vi "太阳能控制器MPPT12.vi"() -> ()   [LabVIEW 2016, in "环境动力监测库.lvlib"]
uses:
  <vilib>/Utility/miscctls.llb/LVPointTypeDef.ctl
  <vilib>/Utility/config.llb/NI_LVConfig.lvlib
  <vilib>/ptbypt/NI_PtbyPt.lvlib
panel:
  out "x+1":u32
  in  "解除告警":bool
  out "串口":string
  in  "串口启用":bool
  in  "MPPT-12 串口":refnum<visa-resource-name> caption="MPPT-12"
  out "状态":string
  out "充放电信息":T1 caption="充放电信息_KWH" {"总累计充电量" format="%.2f"; "当年累计充电量" format="%.2f"; "当月累计充电量" format="%.2f"; "当日累计充电量" format="%.2f"; "当年累计用电量" format="%.2f"; "当月累计用电量" format="%.2f"; "当日累计用电量" format="%.2f"}
  out "通信":bool=TRUE
  out "控制器信息":cluster{"设备温度":dbl}
  out "直流负载信息":cluster{"负载电压":dbl, "负载电流":dbl, "负载功率":dbl}
  out "蓄电池信息":T2
  out "阵列信息":cluster{"阵列电压":dbl, "阵列电流":dbl, "发电功率":dbl}
  # "太阳能控制器MPPT-12"
  # "kW·h"
  # "kW·h"
  # "kW·h"
  # "kW·h"
  # "kW·h"
  # "kW·h"
  # "kW·h"
  # "kW·h"
  # "℃"
  # "V"
  # "A"
  # "W"
  # "V"
  # "A"
  # "V"
  # "V"
  # "℃"
  # "%"
  # "V"
  # "A"
  # "W"
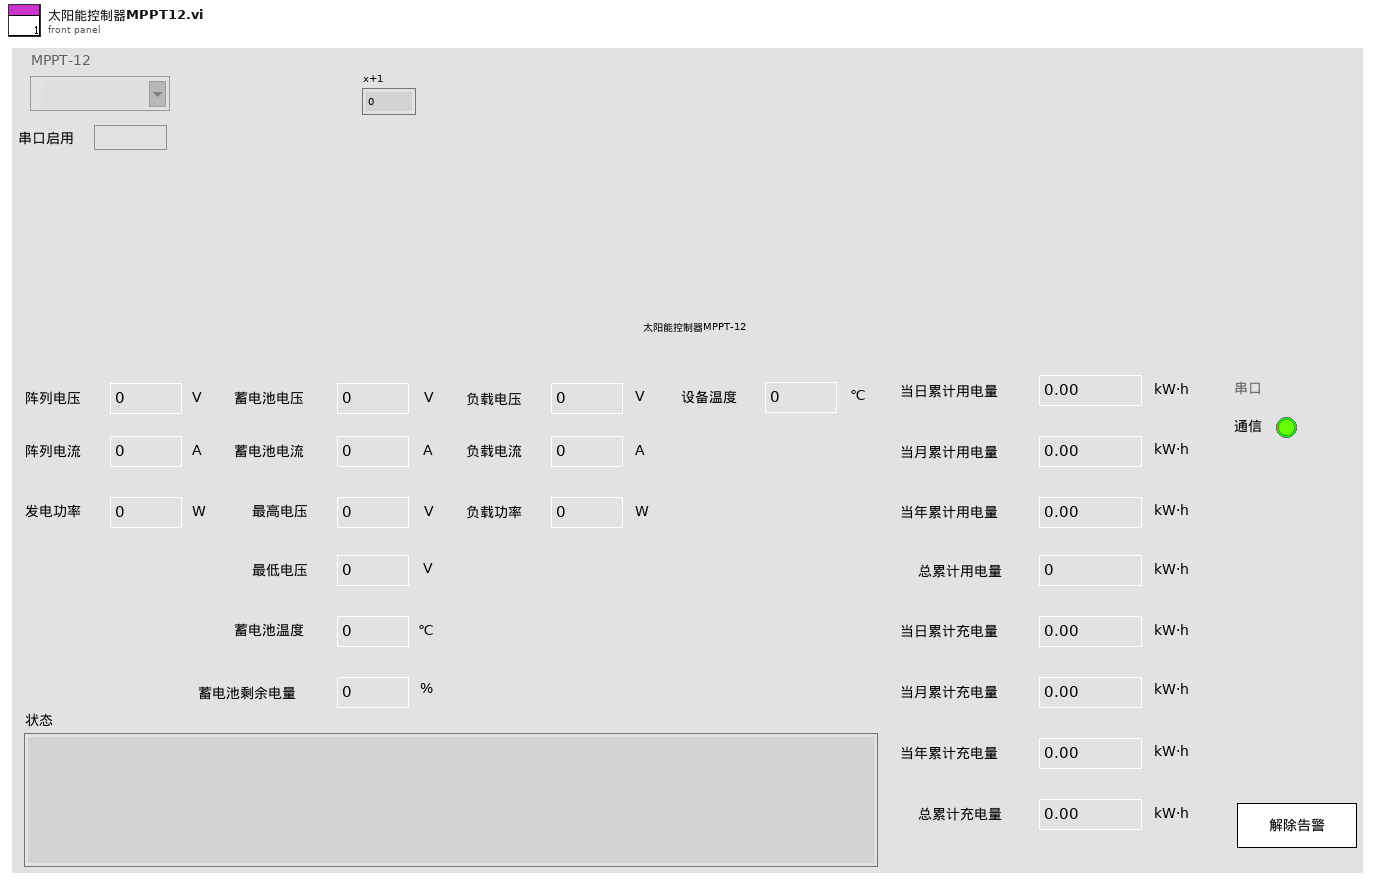
[diagram p1: front panel]
types:
  T1 = cluster{"当日累计用电量":sgl, "当月累计用电量":sgl, "当年累计用电量":sgl, "总累计用电量":sgl, "当日累计充电量":sgl, "当月累计充电量":sgl, "当年累计充电量":sgl, "总累计充电量":sgl}
  T2 = cluster{"蓄电池电压":dbl, "蓄电池电流":dbl, "最高电压":dbl, "最低电压":dbl, "蓄电池温度":dbl, "蓄电池剩余电量":dbl}
  T3 = typedef "LVPointTypeDef.ctl" = cluster{"Horizontal":i16, "Vertical":i16}
  T4 = cluster{"漏水监测输出":cluster{"漏水监测告警":bool, "告警内容":string}, "门禁监测输出":cluster{"门禁监测告警":bool, "告警内容":string}, "门禁监测输出2":cluster{"门禁监测告警":bool, "告警内容":string}, "温湿度监测输出":cluster{"温湿度监测告警":bool, "告警内容":string}, "烟雾监测输出":cluster{"烟雾监测告警":bool, "告警内容":string}, "空调监测输出":cluster{"空调监测告警":bool, "告警内容":string}, "自动重合闸输出":cluster{"自动重合闸告警":bool, "告警内容":string}, "红外入侵输出":cluster{"红外入侵告警":bool, "告警内容":string}, "振动输出":cluster{"振动告警":bool, "告警内容":string}, "UPS输出":cluster{"UPS告警":bool, "告警内容":string}, "蓄电池输出":cluster{"蓄电池告警":bool, "告警内容":string}, "蓄电池输出2":cluster{"蓄电池告警":bool, "告警内容":string}, "GPS输出":cluster{"定位告警":bool, "告警内容":string}, "北斗输出":cluster{"定位告警":bool, "告警内容":string}, "气象输出":cluster{"气象告警":bool, "告警内容":string}, "废液输出":cluster{"废液告警":bool, "告警内容":string}, "废液输出2":cluster{"废液告警":bool, "告警内容":string}}
  T5 = cluster{"时间":timestamp, "阵列电压_V":dbl, "阵列电流_A":dbl, "发电功率_W":dbl, "蓄电池电压_V":dbl, "蓄电池电流_A":dbl, "最高电压_V":dbl, "最低电压_A":dbl, "蓄电池温度_℃":dbl, "蓄电池剩余电量_%":dbl, "负载电压_V":dbl, "负载电流_A":dbl, "负载功率_W":dbl, "设备温度_℃":dbl, "当日累计用电量_KWH":dbl, "当月累计用电量_KWH":dbl, "当年累计用电量_KWH":dbl, "总累计用电量_KWH":dbl, "当日累计充电量_KWH":dbl, "当月累计充电量_KWH":dbl, "当年累计充电量_KWH":dbl, "总累计充电量_KWH":dbl}
  T6 = typedef "LVDateTimeRec.ctl" = cluster{"秒数的小数部分":dbl, "秒":i32, "分":i32, "时":i32, "日":i32, "月":i32, "年":i32, "天数（周）":i32, "天数（年）":i32, "DST":i32}
  T7 = cluster{"市电":cluster{"状态":bool, "电压:":u16, "电流：":dbl, "详情  ":bool}, "UPS":cluster{"状态":bool, "输入电压:":sgl, "输出电压:":sgl, "电池电量:":u8, "电量":u16, "详情  ":bool}, "蓄电池12V":cluster{"状态":bool, "电压:":sgl, "电流:":sgl, "电池电量:":u8, "电量":u16, "详情  ":bool, "充电":bool, "负载":bool}, "蓄电池24V":cluster{"状态":bool, "电压:":sgl, "电流:":sgl, "电池电量:":u8, "电量":u16, "详情  ":bool, "充电":bool, "负载":bool}}
  T8 = cluster{"状态":cluster{"蓄电池状态":string, "阵列状态":string, "充电状态":string, "负载状态":string, "设备状态":string}, "充放电信息":cluster{"当日累计用电量":sgl, "当月累计用电量":sgl, "当年累计用电量":sgl, "总累计用电量":sgl, "当日累计充电量":sgl, "当月累计充电量":sgl, "当年累计充电量":sgl, "总累计充电量":sgl}, "控制器信息":cluster{"设备温度℃":dbl}, "蓄电池信息":cluster{"蓄电池电压V":dbl, "蓄电池电流A":dbl, "最高电压V":dbl, "最低电压A":dbl, "蓄电池温度℃":dbl, "蓄电池剩余电量%":dbl}, "阵列信息":cluster{"阵列电压V":dbl, "阵列电流A":dbl, "发电功率W":dbl}, "直流负载信息":cluster{"负载电压V":dbl, "负载电流A":dbl, "负载功率W":dbl}, "error out":errorcluster}
  T9 = enum32{"Bad", "Idle", "Run top level", "Running"}
  T10 = typedef "NI_LVConfig.lvlib/Config Data RefNum.ctl" = refnum<k1>
  T11 = enum8{"Enabled", "Disabled", "Disabled and Grayed Out"}
  T12 = cluster{"蓄电池电压V":dbl, "蓄电池电流A":dbl, "最高电压V":dbl, "最低电压A":dbl, "蓄电池温度℃":dbl, "蓄电池剩余电量%":dbl}
  T13 = cluster{"蓄电池状态":string, "阵列状态":string, "充电状态":string, "负载状态":string, "设备状态":string}
  T14 = cluster{"baud rate (bps)":u32, "stop bits":u16, "parity":u16, "flow control":u16, "timeout":u32, "retries":i32}
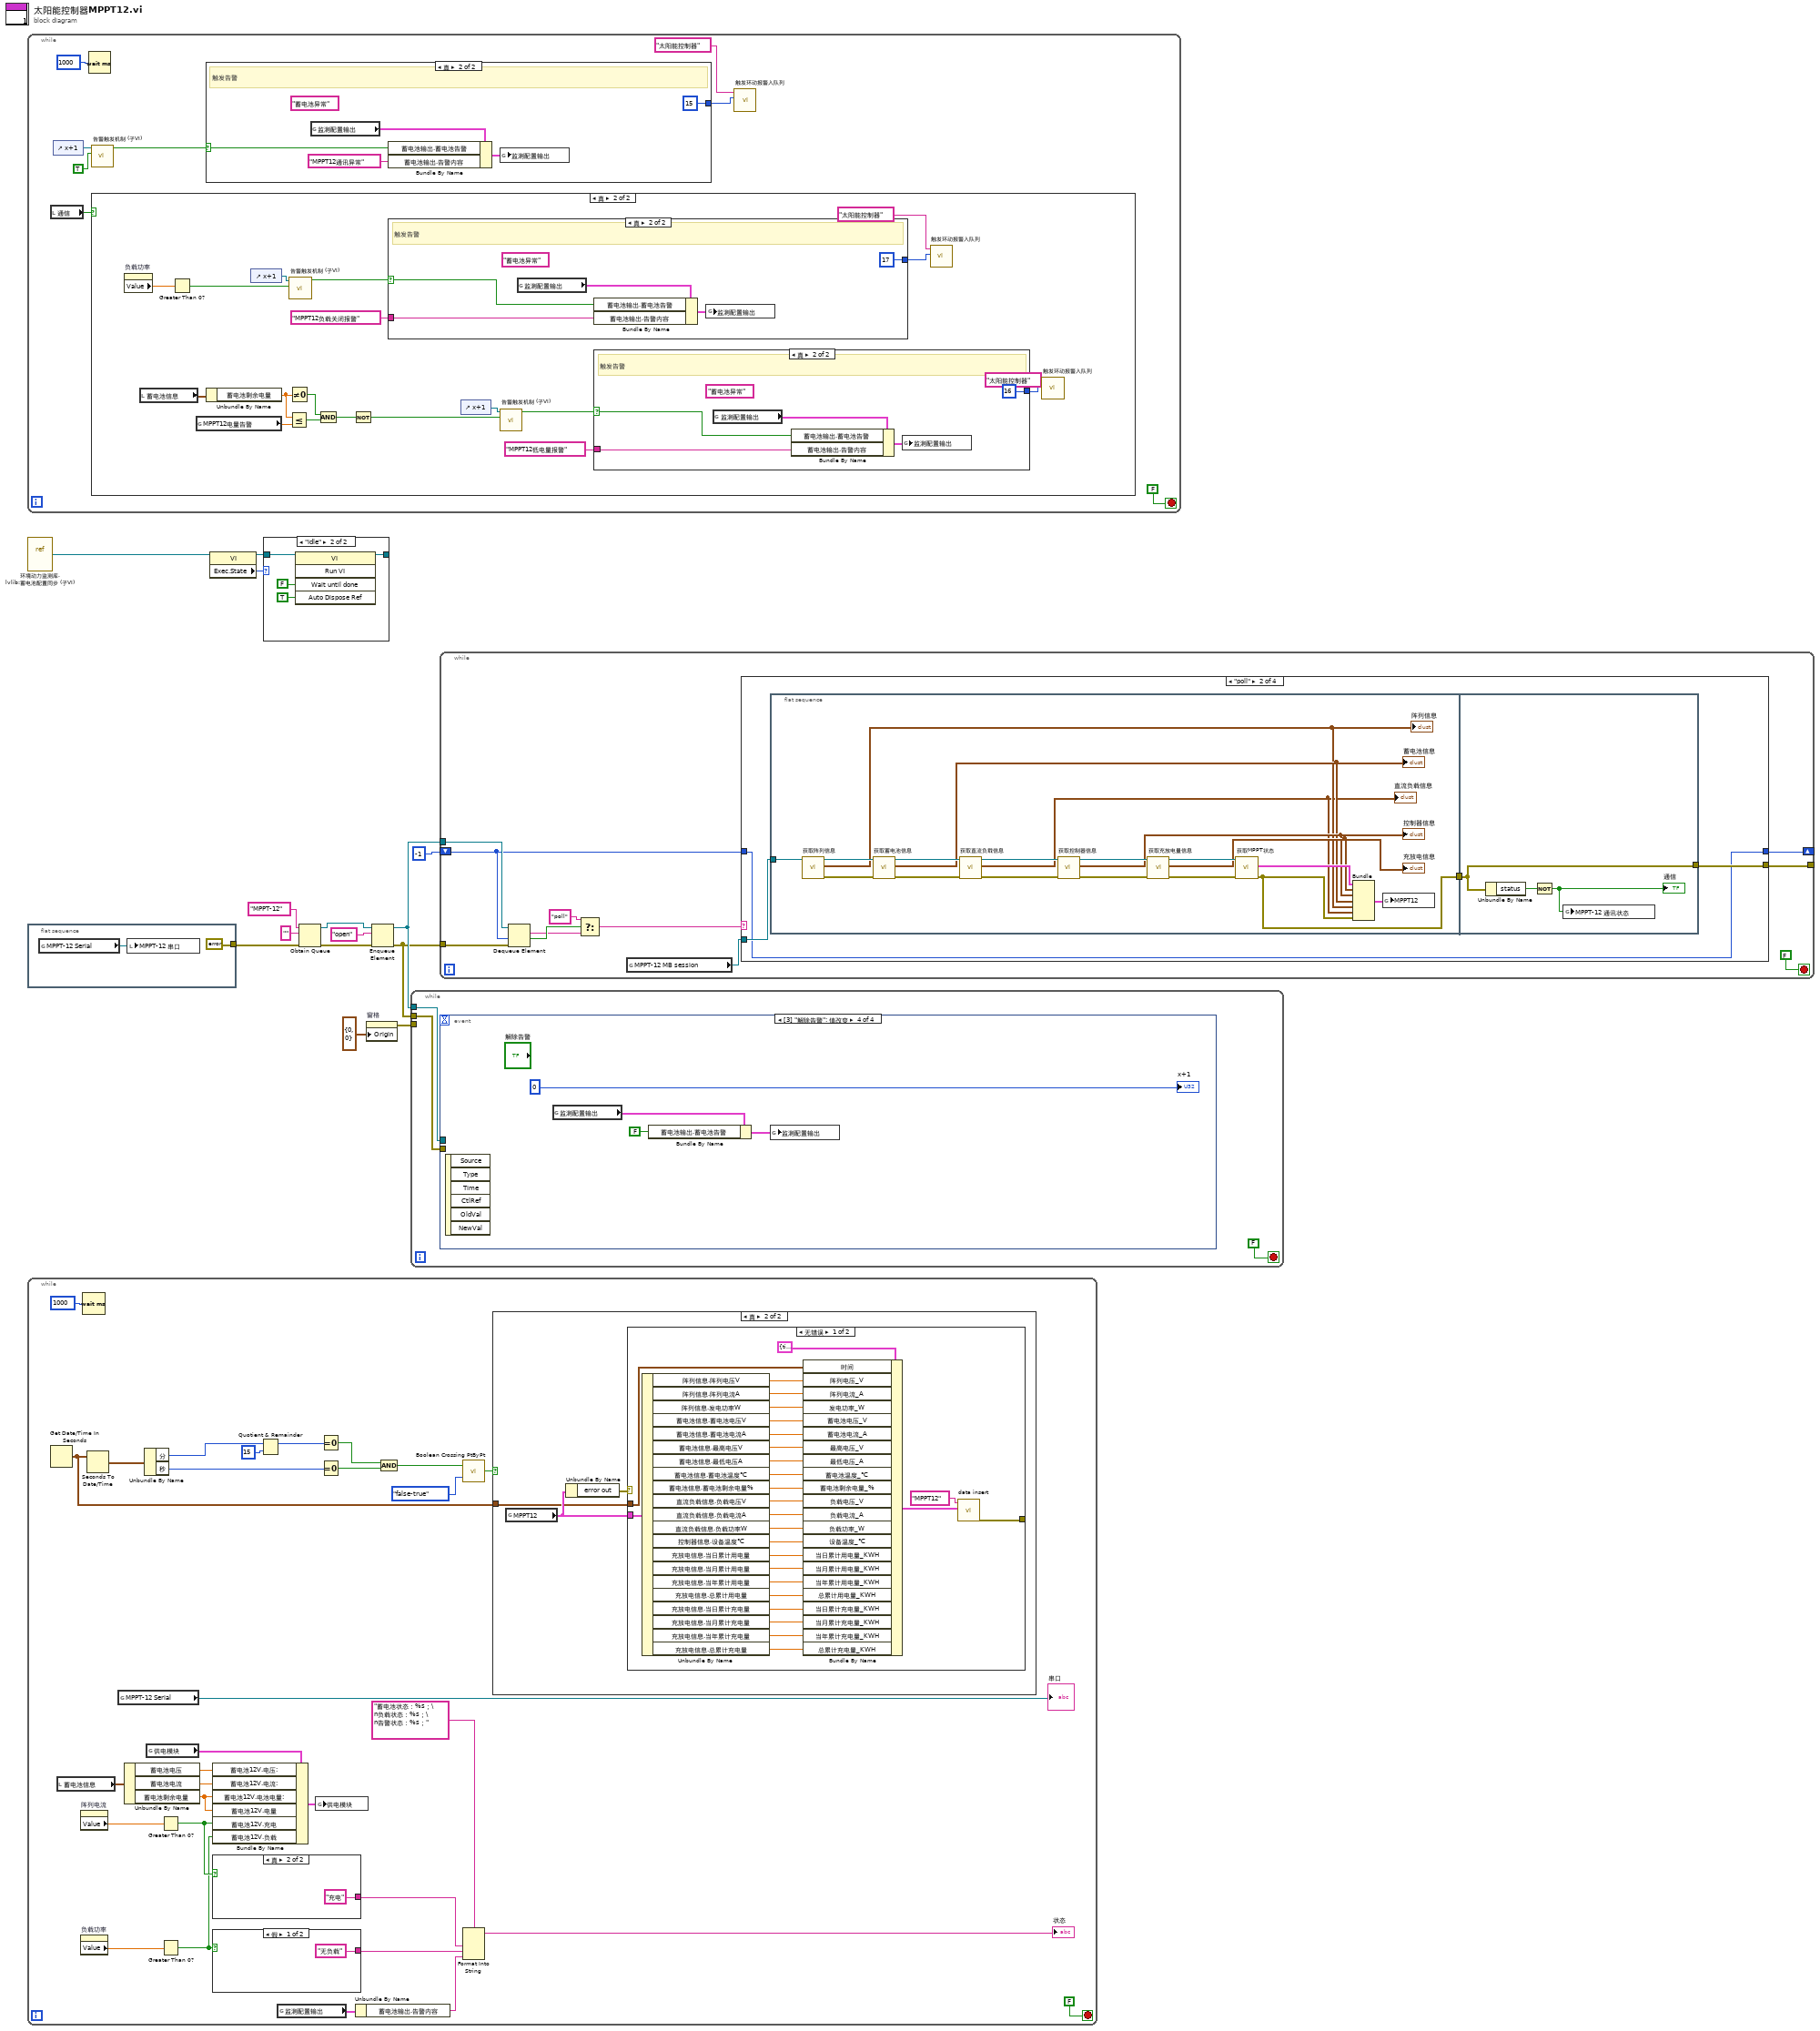
[diagram p0: block diagram]
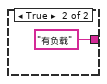
[diagram p7: hidden frame]
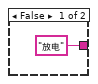
[diagram p8: hidden frame]
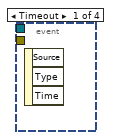
[diagram p11: hidden frame]
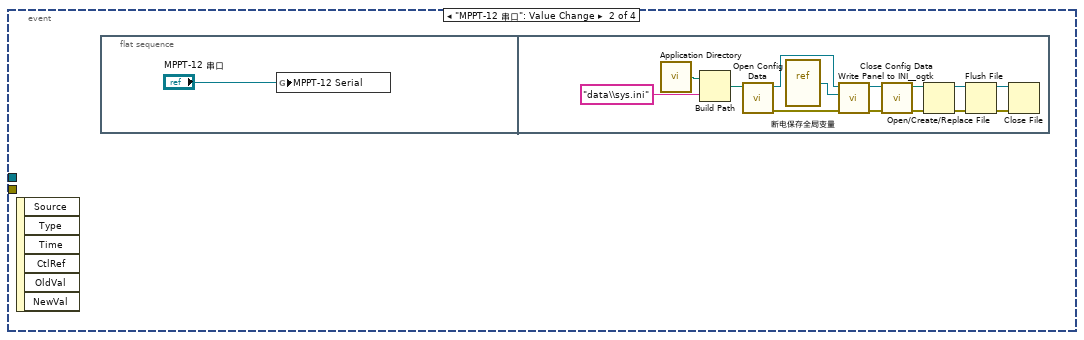
[diagram p12: hidden frame]
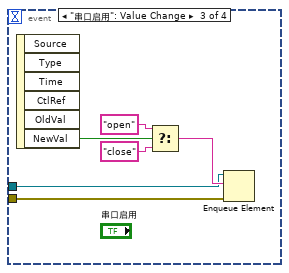
[diagram p13: hidden frame]
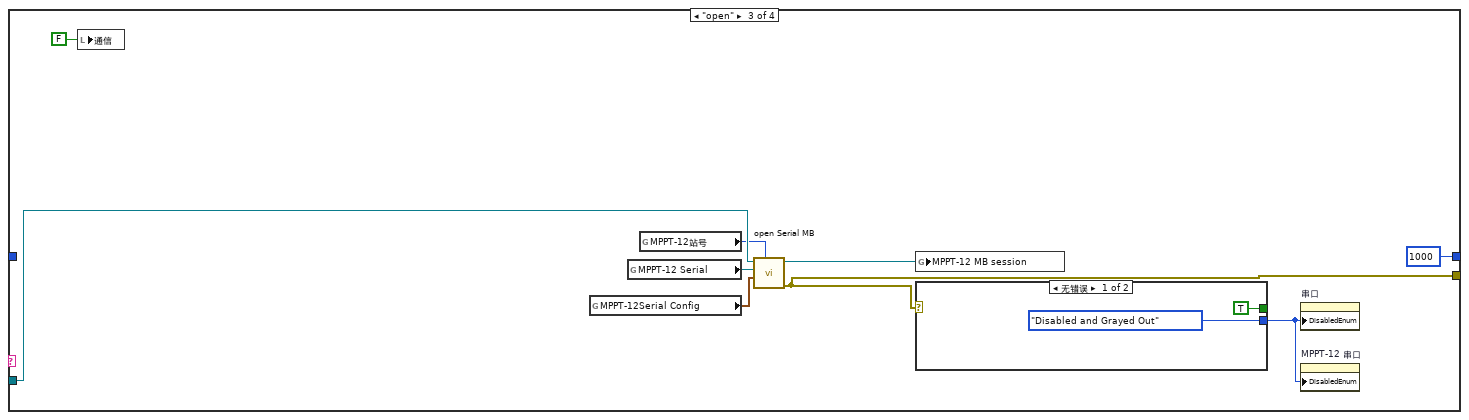
[diagram p15: hidden frame]
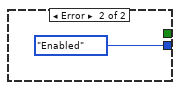
[diagram p16: hidden frame]
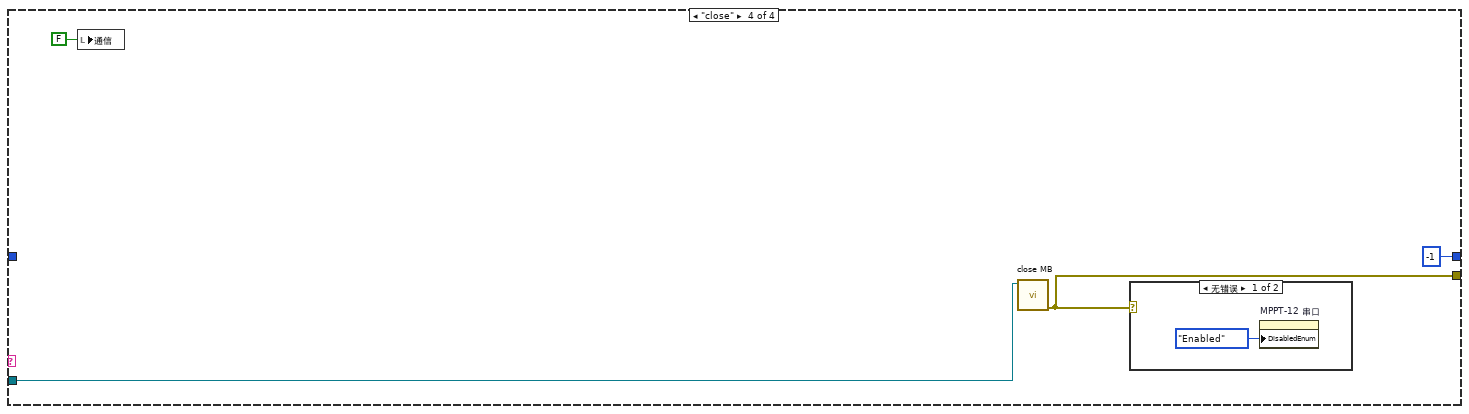
[diagram p17: hidden frame]
diagram:
  n1 = while {
    stop <- FALSE stop-if-true
    n2 = local read "通信"() -> (w20:bool)
    n3 = control-ref of="x+1"() -> (w19:refnum<vi>)
    n4 = Wait (ms)(milliseconds to wait=u32 1000 ("等待时间（毫秒）")) -> ()  [unwired: 1 out]
    n5 = call "告警触发机制 (子VI).vi"("状态输出"=TRUE, "Digital输入"=w19) -> ("触发告警"=w18:bool)  [unwired: 8 in, 1 out]
    n6 = case shown="真" w20 {
      frame False {
      }
      frame True {
        n7 = property on="负载功率" class="DigNum (严格)"() -> ("Value"=w36:dbl)  [unwired: 2 in, 2 out]
        n8 = local read "蓄电池信息"() -> (w46:T2)
        n9 = Greater Than 0?(x=w36) -> (x > 0?=w34:bool)
        n10 = global read "断电保存全局变量.vi" "MPPT12电量告警"() -> (w45:dbl)
        n11 = Unbundle By Name(w46) -> ("蓄电池剩余电量"=w39:dbl)
        n12 = control-ref of="x+1"() -> (w35:refnum<vi>)
        n13 = Less Or Equal?(x=w39, y=w45) -> (x <= y?=w40:bool)
        n14 = Not Equal To 0?(x=w39) -> (x != 0?=w38:bool)
        n15 = call "告警触发机制 (子VI).vi"("状态输出"=w34, "Digital输入"=w35) -> ("触发告警"=w32:bool)  [unwired: 8 in, 1 out]
        n16 = And(x=w38, y=w40) -> (x .and. y?=w37:bool)
        n17 = Not(x=w37) -> (.not. x?=w43:bool)
        n18 = case shown="真" w32 {
          selector: w32 -> [_ w51]
          tunnel: "MPPT12负载关闭报警" ("设备") -> [_ w48]
          tunnel: [_ 17 ("code")] -> w29
          frame False {
          }
          frame True {
            (unwired) "蓄电池异常" ("设备")
            # "触发告警"
            n19 = global read "内部交互全局变量.vi" "监测配置输出"() -> (w50:T4)
            n20 = Bundle By Name(cluster=w50, "蓄电池输出.蓄电池告警"=w51, "蓄电池输出.告警内容"=w48) -> (w49:T4)
            n21 = global write "内部交互全局变量.vi" "监测配置输出"(w49) -> ()
          }
        }
        n22 = control-ref of="x+1"() -> (w41:refnum<vi>)
        n23 = call "告警触发机制 (子VI).vi"("状态输出"=w43, "Digital输入"=w41) -> ("触发告警"=w42:bool)  [unwired: 8 in, 1 out]
        n24 = case shown="真" w42 {
          selector: w42 -> [_ w56]
          tunnel: "MPPT12低电量报警" ("设备") -> [_ w53]
          tunnel: [_ 16 ("code")] -> w31
          frame False {
          }
          frame True {
            (unwired) "蓄电池异常" ("设备")
            # "触发告警"
            n25 = global read "内部交互全局变量.vi" "监测配置输出"() -> (w55:T4)
            n26 = Bundle By Name(cluster=w55, "蓄电池输出.蓄电池告警"=w56, "蓄电池输出.告警内容"=w53) -> (w54:T4)
            n27 = global write "内部交互全局变量.vi" "监测配置输出"(w54) -> ()
          }
        }
        n28 = call "触发环动报警入队列.vi"("code"=w29, "元器件"="太阳能控制器") -> ()  [unwired: 10 in]
        n29 = call "触发环动报警入队列.vi"("code"=w31, "元器件"="太阳能控制器") -> ()  [unwired: 10 in]
      }
    }
    n30 = case shown="真" w18 {
      selector: w18 -> [_ w27]
      tunnel: [_ 15 ("code")] -> w15
      frame False {
      }
      frame True {
        (unwired) "蓄电池异常" ("设备")
        # "触发告警"
        n31 = global read "内部交互全局变量.vi" "监测配置输出"() -> (w26:T4)
        n32 = Bundle By Name(cluster=w26, "蓄电池输出.蓄电池告警"=w27, "蓄电池输出.告警内容"="MPPT12通讯异常" ("报警内容")) -> (w25:T4)
        n33 = global write "内部交互全局变量.vi" "监测配置输出"(w25) -> ()
      }
    }
    n34 = call "触发环动报警入队列.vi"("code"=w15, "元器件"="太阳能控制器") -> ()  [unwired: 10 in]
  }
  n35 = vi-ref "环境动力监测库.lvlib:蓄电池配置同步 (子VI).vi"() -> (w2:refnum<vi>)
  n36 = flat-sequence {
    tunnel: [errorcluster {"status"=FALSE, "code"=0, "source"=""} ("error out")] -> w1
    frame #0 {
      n37 = global read "断电保存全局变量.vi" "MPPT-12 Serial"() -> (w58:refnum<visa-resource-name>)
      n38 = local write "MPPT-12 串口"(w58) -> ()
    }
  }
  n39 = while {
    stop <- FALSE stop-if-true
    n40 = Get Date/Time In Seconds() -> (seconds since 1Jan1904=w76:timestamp)
    n41 = local read "蓄电池信息"() -> (w72:T2)
    n42 = property on="阵列电流" class="DigNum (严格)"() -> ("Value"=w67:dbl)  [unwired: 2 in, 2 out]
    n43 = property on="负载功率" class="DigNum (严格)"() -> ("Value"=w63:dbl)  [unwired: 2 in, 2 out]
    n44 = Wait (ms)(milliseconds to wait=u32 1000 ("等待时间（毫秒）")) -> ()  [unwired: 1 out]
    n45 = Seconds To Date/Time(time stamp (now)=w76) -> (date time rec=w86:T6)  [unwired: 1 in]
    n46 = global read "断电保存全局变量.vi" "MPPT-12 Serial"() -> (→"串口":refnum<visa-resource-name>)
    n47 = Unbundle By Name(w72) -> ("蓄电池电压"=w71:dbl, "蓄电池电流"=w70:dbl, "蓄电池剩余电量"=w69:dbl)
    n48 = Unbundle By Name(w86) -> ("分"=w85:i32, "秒"=w82:i32)
    n49 = global read "内部交互全局变量.vi" "供电模块"() -> (w74:T7)
    n50 = Greater Than 0?(x=w67) -> (x > 0?=w64:bool)
    n51 = Greater Than 0?(x=w63) -> (x > 0?=w59:bool)
    n52 = Bundle By Name(cluster=w74, "蓄电池12V.电压:"=w71, "蓄电池12V.电流:"=w70, "蓄电池12V.电池电量:"=w69, "蓄电池12V.电量"=w69, "蓄电池12V.充电"=w64, "蓄电池12V.负载"=w59) -> (w73:T7)
    n53 = case shown="真" w64 {
      tunnel: ["放电" "充电"] -> w66
      frame False {
      }
      frame True {
      }
    }
    n54 = case shown="假" w59 {
      tunnel: ["无负载" "有负载"] -> w62
      frame False {
      }
      frame True {
      }
    }
    n55 = Quotient & Remainder(x=w85, y=15) -> (x-y*floor(x/y)=w83:i32)  [unwired: 1 out]
    n56 = global read "内部交互全局变量.vi" "监测配置输出"() -> (w61:T4)
    n57 = global write "内部交互全局变量.vi" "供电模块"(w73) -> ()
    n58 = Equal To 0?(x=w83) -> (x = 0?=w81:bool)
    n59 = Equal To 0?(x=w82) -> (x = 0?=w80:bool)
    n60 = Unbundle By Name(w61) -> ("蓄电池输出.告警内容"=w60:string)
    n61 = And(x=w81, y=w80) -> (x .and. y?=w79:bool)
    n62 = call <vilib>:"Boolean Crossing PtByPt.vi"("direction"=enum16{"either", "false-true", "true-false"}."false-true", "input"=w79) -> ("crossing"=w77:bool)  [unwired: 1 in]
    n63 = Format Into String(format string="蓄电池状态：%s；\n负载状态：%s；\n告警状态：%s；" ("格式字符串"), w66, w62, w60) -> (resulting string=→"状态":string)  [unwired: 2 in, 1 out]
    n64 = case shown="真" w77 {
      tunnel: w76 -> [_ w93]
      frame False {
      }
      frame True {
        n65 = global read "太阳能控制器全局.vi" "MPPT12"() -> (w94:T8)
        n66 = Unbundle By Name(w94) -> ("error out"=w95:errorcluster)
        n67 = case shown="无错误" w95 {
          tunnel: w94 -> [w100 _]
          tunnel: w93 -> [w99 _]
          tunnel: [w96 _] -> _
          frame No Error {
            n68 = Unbundle By Name(w100) -> ("阵列信息.阵列电压V"=w102:dbl, "阵列信息.阵列电流A"=w103:dbl, "阵列信息.发电功率W"=w104:dbl, "蓄电池信息.蓄电池电压V"=w105:dbl, "蓄电池信息.蓄电池电流A"=w106:dbl, "蓄电池信息.最高电压V"=w107:dbl, "蓄电池信息.最低电压A"=w108:dbl, "蓄电池信息.蓄电池温度℃"=w109:dbl, "蓄电池信息.蓄电池剩余电量%"=w110:dbl, "直流负载信息.负载电压V"=w111:dbl, "直流负载信息.负载电流A"=w112:dbl, "直流负载信息.负载功率W"=w113:dbl, "控制器信息.设备温度℃"=w114:dbl, "充放电信息.当日累计用电量"=w115:sgl, "充放电信息.当月累计用电量"=w116:sgl, "充放电信息.当年累计用电量"=w117:sgl, "充放电信息.总累计用电量"=w118:sgl, "充放电信息.当日累计充电量"=w119:sgl, "充放电信息.当月累计充电量"=w120:sgl, "充放电信息.当年累计充电量"=w121:sgl, "充放电信息.总累计充电量"=w122:sgl)
            n69 = Bundle By Name(cluster=T5 {"时间"=timestamp(0 s since 1904-01-01), "阵列电压_V"=0.0, "阵列电流_A"=0.0, "发电功率_W"=0.0, "蓄电池电压_V"=0.0, "蓄电池电流_A"=0.0, "最高电压_V"=0.0, "最低电压_A"=0.0, "蓄电池温度_℃"=0.0, "蓄电池剩余电量_%"=0.0, "负载电压_V"=0.0, "负载电流_A"=0.0, "负载功率_W"=0.0, "设备温度_℃"=0.0, "当日累计用电量_KWH"=0.0, "当月累计用电量_KWH"=0.0, "当年累计用电量_KWH"=0.0, "总累计用电量_KWH"=0.0, "当日累计充电量_KWH"=0.0, "当月累计充电量_KWH"=0.0, "当年累计充电量_KWH"=0.0, "总累计充电量_KWH"=0.0} ("data in"), "时间"=w99, "阵列电压_V"=w102, "阵列电流_A"=w103, "发电功率_W"=w104, "蓄电池电压_V"=w105, "蓄电池电流_A"=w106, "最高电压_V"=w107, "最低电压_A"=w108, "蓄电池温度_℃"=w109, "蓄电池剩余电量_%"=w110, "负载电压_V"=w111, "负载电流_A"=w112, "负载功率_W"=w113, "设备温度_℃"=w114, "当日累计用电量_KWH"=w115, "当月累计用电量_KWH"=w116, "当年累计用电量_KWH"=w117, "总累计用电量_KWH"=w118, "当日累计充电量_KWH"=w119, "当月累计充电量_KWH"=w120, "当年累计充电量_KWH"=w121, "总累计充电量_KWH"=w122) -> (w98:T5)
            n70 = call "data insert.vi"("data in"=w98, "table"="MPPT12") -> ("error out"=w96:errorcluster)  [unwired: 9 in]
          }
          frame Error {
          }
        }
      }
    }
  }
  n71 = property class="VI"(reference=w2) -> (reference out=w3:refnum<vi>, "Exec.State"=w4:T9)  [unwired: 1 in, 1 out]
  n72 = case shown="\"Idle\"" w4 {
    tunnel: w3 -> [w123 w125]
    tunnel: [w123 w124] -> _
    frame "Bad", Default {
    }
    frame "Idle" {
      n73 = invoke class="VI" method="Run VI"(reference=w125, "Wait until done"=FALSE ("结束前等待"), "Auto Dispose Ref"=TRUE ("自动销毁引用")) -> (reference out=w124:refnum<vi>)  [unwired: 2 in, 4 out]
    }
  }
  n74 = Obtain Queue(name (unnamed)="MPPT-12" ("名称（未命名）"), element data type="", error in (no error)=w1) -> (queue out=w8:refnum<queue>, error out=w7:errorcluster)  [unwired: 2 in, 1 out]
  n75 = property on="窗格" class="Pane"("Origin"=T3 {"Horizontal"=0, "Vertical"=0} ("原点")) -> (error out=w12:errorcluster)  [unwired: 2 in, 1 out]
  n76 = Enqueue Element(queue=w8, element="open" ("元素"), error in (no error)=w7) -> (queue out=w6:refnum<queue>, error out=w5:errorcluster)  [unwired: 1 in, 1 out]
  n77 = while {
    tunnel: w12 -> [_]
    tunnel: w6 -> [w129]
    tunnel: w5 -> [w128]
    stop <- FALSE stop-if-true
    n78 = event shown="[3] \"解除告警\": 值改变" {
      selector: _ -> [_ _ _ _]
      dyn-events: _ -> [_ _ _ _]
      timeout: _ -> [_ _ _ _]
      tunnel: w129 -> [_ _ w147 _]
      tunnel: w128 -> [_ _ w146 _]
      event Timeout {
        n79 = event-data() -> ()  [unwired: 1 in, 3 out]
      }
      event "MPPT-12 串口": Value Change {
        n80 = event-data() -> ()  [unwired: 1 in, 6 out]
        n81 = flat-sequence {
          frame #0 {
            n82 = global write "断电保存全局变量.vi" "MPPT-12 Serial"("MPPT-12 串口") -> ()
          }
          frame #1 {
            n83 = call <vilib>:"Application Directory.vi"() -> ("Application Directory"=w145:path)
            n84 = Build Path(base path=w145, name or relative path="data\\sys.ini" ("名称或相对路径")) -> (appended path=w143:path)
            n85 = call <vilib>:"Open Config Data.vi"("configuration file path"=w143) -> ("error out"=w139:errorcluster, "refnum"=w142:T10)  [unwired: 8 in, 1 out]
            n86 = vi-ref "断电保存全局变量.vi"() -> (w141:refnum<vi>)
            n87 = call <userlib>:"Write Panel to INI__ogtk.vi"("error in (no error)"=w139, "VI ref"=w141, "refnum"=w142) -> ("error out"=w138:errorcluster, "refnum out"=w140:T10)  [unwired: 7 in]
            n88 = call <vilib>:"Close Config Data.vi"("error in (no error)"=w138, "refnum"=w140) -> ("error out"=w133:errorcluster, "file path"=w132:path)  [unwired: 8 in]
            n89 = Open/Create/Replace File(file path (use dialog)=w132, error in=w133) -> (refnum out=w136:refnum<file>, error out=w137:errorcluster)  [unwired: 4 in, 1 out]
            n90 = Flush File(refnum=w136, error in=w137) -> (refnum out=w135:refnum<file>, error out=w134:errorcluster)
            n91 = Close File(refnum=w135, error in=w134) -> ()  [unwired: 2 out]
          }
        }
      }
      event "串口启用": Value Change {
        n92 = event-data() -> ("NewVal"=w148:bool)  [unwired: 1 in, 5 out]
        n93 = Select(t="open", s=w148, f="close") -> (s? t:f=w150:string)
        n94 = Enqueue Element(queue=w147, element=w150, error in (no error)=w146) -> ()  [unwired: 1 in, 3 out]
      }
      event "解除告警": Value Change {
        n95 = event-data() -> ()  [unwired: 1 in, 6 out]
        n96 = global read "内部交互全局变量.vi" "监测配置输出"() -> (w153:T4)
        n97 = Bundle By Name(cluster=w153, "蓄电池输出.蓄电池告警"=FALSE) -> (w152:T4)
        n98 = global write "内部交互全局变量.vi" "监测配置输出"(w152) -> ()
        "x+1" <- u32 0 ("x+1")
      }
    }
  }
  n99 = while {
    shift-right: [w157] -> _
    shift-left: -1 ("超时毫秒(-1)") -> [w158]
    tunnel: w6 -> [w163]
    tunnel: [w159] -> _
    tunnel: w5 -> [w156]
    stop <- FALSE stop-if-true
    n100 = Dequeue Element(queue=w163, timeout in ms (-1)=w158, error in (no error)=w156) -> (element=w164:string, timed out?=w166:bool)  [unwired: 2 out]
    n101 = Select(t="poll" ("元素"), s=w166, f=w164) -> (s? t:f=w161:string)
    n102 = global read "太阳能控制器全局.vi" "MPPT-12 MB session"() -> (w160:refnum<class "MB_Master.lvclass">)
    n103 = case shown="\"poll\"" w161 {
      tunnel: w160 -> [_ w171 w201 w208]
      tunnel: [_ w169 w199 w206] -> w159
      tunnel: w158 -> [w167 w168 _ _]
      tunnel: [w167 w168 1000 ("超时毫秒(-1)") -1 ("超时毫秒(-1)")] -> w157
      frame Default {
      }
      frame "poll" {
        n104 = flat-sequence {
          tunnel: w171 -> [w190]
          tunnel: [w173] -> w170
          tunnel: w170 -> [w191]
          tunnel: [w191] -> w169
          frame #0 {
            n105 = call "获取阵列信息.vi"("MB session in"=w190) -> ("error out"=w188:errorcluster, "阵列信息"=w175:cluster{"阵列电压V":dbl, "阵列电流A":dbl, "发电功率W":dbl}, "MB session out"=w189:refnum<class "MB_Master.lvclass">)  [unwired: 8 in]
            "阵列信息" <- w175
            n106 = call "获取蓄电池信息.vi"("error in (no error)"=w188, "MB session in"=w189) -> ("error out"=w186:errorcluster, "蓄电池信息"=w176:T12, "MB session out"=w187:refnum<class "MB_Master.lvclass">)  [unwired: 7 in]
            "蓄电池信息" <- w176
            n107 = call "获取直流负载信息.vi"("error in (no error)"=w186, "MB session in"=w187) -> ("error out"=w184:errorcluster, "直流负载信息"=w174:cluster{"负载电压V":dbl, "负载电流A":dbl, "负载功率W":dbl}, "MB session out"=w185:refnum<class "MB_Master.lvclass">)  [unwired: 7 in]
            "直流负载信息" <- w174
            n108 = call "获取控制器信息.vi"("error in (no error)"=w184, "MB session in"=w185) -> ("error out"=w182:errorcluster, "控制器信息"=w177:cluster{"设备温度℃":dbl}, "MB session out"=w183:refnum<class "MB_Master.lvclass">)  [unwired: 7 in]
            "控制器信息" <- w177
            n109 = call "获取充放电量信息.vi"("error in (no error)"=w182, "MB session in"=w183) -> ("error out"=w180:errorcluster, "充放电信息"=w178:T1, "MB session out"=w181:refnum<class "MB_Master.lvclass">)  [unwired: 7 in]
            "充放电信息" <- w178
            n110 = call "获取MPPT状态.vi"("error in (no error)"=w180, "MB session in"=w181) -> ("error out"=w173:errorcluster, "状态"=w179:T13)  [unwired: 6 in, 2 out]
            n111 = Bundle("状态"=w179, "充放电信息"=w178, "控制器信息"=w177, "蓄电池信息"=w176, "阵列信息"=w175, "直流负载信息"=w174, "error out"=w173) -> (w172:T8)  [unwired: 1 in]
            n112 = global write "太阳能控制器全局.vi" "MPPT12"(w172) -> ()
          }
          frame #1 {
            n113 = Unbundle By Name(w191) -> ("status"=w193:bool)
            n114 = Not(x=w193) -> (.not. x?=w192:bool)
            "通信" <- w192
            n115 = global write "太阳能控制器全局.vi" "MPPT-12 通讯状态"(w192) -> ()
          }
        }
      }
      frame "open" {
        n116 = local write "通信"(FALSE ("通讯状态 2")) -> ()
        n117 = global read "断电保存全局变量.vi" "MPPT-12Serial Config"() -> (w194:T14)
        n118 = global read "断电保存全局变量.vi" "MPPT-12 Serial"() -> (w197:refnum<visa-resource-name>)
        n119 = global read "断电保存全局变量.vi" "MPPT-12站号"() -> (w195:u64)
        n120 = call "open Serial MB.vi"("Slave ID"=w195, "Serial Config"=w194, "VISA Resource"=w197, "MB session in"=w201) -> ("error out"=w199:errorcluster, "MB session out"=w200:refnum<class "MB_Master.lvclass">)  [unwired: 6 in]
        n121 = global write "太阳能控制器全局.vi" "MPPT-12 MB session"(w200) -> ()
        n122 = case shown="无错误" w199 {
          tunnel: [T11."Disabled and Grayed Out" ("禁用") T11."Enabled" ("禁用")] -> w196
          tunnel: [TRUE _] -> _
          frame No Error {
          }
          frame Error {
          }
        }
        n123 = property on="串口" class="Str"("DisabledEnum"=w196) -> ()  [unwired: 2 in, 2 out]
        n124 = property on="MPPT-12 串口" class="VISAName"("DisabledEnum"=w196) -> ()  [unwired: 2 in, 2 out]
      }
      frame "close" {
        n125 = local write "通信"(FALSE ("通讯状态 2")) -> ()
        n126 = call "close MB.vi"("MB session in"=w208) -> ("error out"=w206:errorcluster)  [unwired: 10 in]
        n127 = case shown="无错误" w206 {
          frame No Error {
            n128 = property on="MPPT-12 串口" class="VISAName"("DisabledEnum"=T11."Enabled" ("禁用")) -> ()  [unwired: 2 in, 2 out]
          }
          frame Error {
          }
        }
      }
    }
  }
